vi "Noise Synthesis Test.vi"() -> ()   [LabVIEW 2015]
uses:
  Controls/Level XCtl/Level XCtl.xctl
  <vilib>/Analysis/5stat.llb/RMS (DBL).vi
  Top Level VIs/Stimulus-Set Level.vi
  Utility VIs/Math VIs/Linear to dB (scalar).vi
  Utility VIs/Math VIs/FFT x(t) to dB,Degrees (1D).vi
  <vilib>/Analysis/NI_AALPro.lvlib
panel:
  out "dB Vrms":dbl
  in  "Level":T2(xcontrol) caption="Level XCtl"
  in  "Slope Fmin (Hz)":dbl=500.0
  out "XY Graph":cluster{"Array":dbl[], "Array":dbl[]}(graph)
  out "Waveform Graph":dbl[](graph)
  out "error out":errorcluster
  in  "error in (no error)":errorcluster
  in  "Length (points)":i32=100000
  in  "Sampling rate (Hz)":dbl=50000.0
  in  "Max Frequency (Hz)":dbl=1000.0
  in  "Slope (dB/oct)":dbl=-3.0
  in  "Min Frequency (Hz)":dbl=100.0
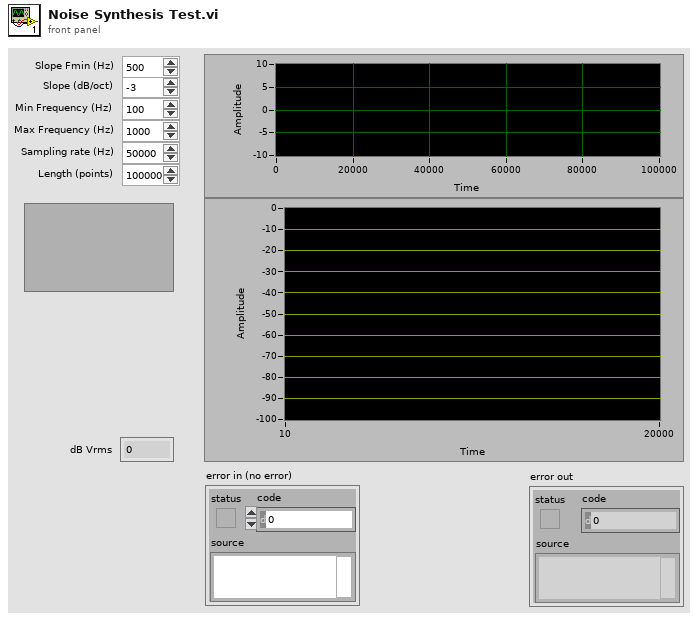
[diagram p1: front panel]
types:
  T1 = typedef "Level Units.ctl" = enum16{"dB atten", "dB SPL", "dB re 1 Vrms", "dB V/Hz½", "mW", "dB HL", "Volts", "dB mW"}
  T2 = cluster{"Level":dbl, "Units":T1, "Max":dbl, "Multiplier":dbl, "Cal File":path, "Cal":cluster{"Freq (Hz)":dbl[], "Mag (dB SPL)":dbl[], "Phase (deg)":dbl[]}}
  T3 = cluster{"Level":dbl, "Mode":T1, "Max":dbl, "Multiplier":dbl, "Cal File":path, "Cal":cluster{"Freq (Hz)":dbl[], "Mag (dB SPL)":dbl[], "Phase (deg)":dbl[]}}
  T4 = typedef "Level XCtl.xctl/Level Data.ctl" = cluster{"Level":dbl, "Units":T1, "Max":dbl, "Multiplier":dbl, "Cal File":path, "Cal":cluster{"Freq (Hz)":dbl[], "Mag (dB SPL)":dbl[], "Phase (deg)":dbl[]}}
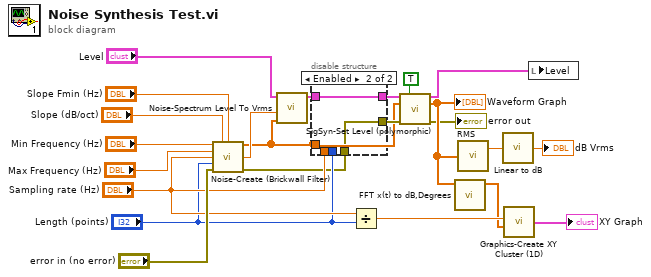
[diagram p0: block diagram]
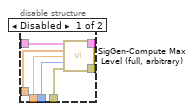
[diagram p2: hidden frame]
diagram:
  n1 = call "Noise-Create (Brickwall Filter).vi"("Min Frequency (Hz)"="Min Frequency (Hz)", "Slope (dB/oct)"="Slope (dB/oct)", "Slope Fmin (Hz)"="Slope Fmin (Hz)", "Max Frequency (Hz)"="Max Frequency (Hz)", "Sampling rate (Hz)"="Sampling rate (Hz)", "Length (points)"="Length (points)", "error in (no error)"="error in (no error)") -> ("Filtered Noise"=w2:dbl[], "dB Vrms of spectrum level = 0"=w14:dbl, "error out"=w4:errorcluster)  [unwired: 6 in]
  n2 = call "Noise-Spectrum Level To Vrms.vi"("Filtered Noise"=w2, "dB Vrms of spectrum level = 0"=w14, "Level In"="Level") -> ("Level Out"=w12:T3)  [unwired: 7 in, 1 out]
  n3 = disable-structure shown="Enabled" {
    disable-tunnel: w12 -> [w30 w32]
    disable-tunnel: [w29 w32] -> w11
    disable-tunnel: "Sampling rate (Hz)" -> [w28 _]
    disable-tunnel: "Length (points)" -> [w27 _]
    disable-tunnel: [w26 w31] -> w5
    disable-tunnel: w4 -> [w25 w31]
    disable-tunnel: w2 -> [w24 _]
    frame Disabled {
      n4 = call "SigGen-Compute Max Level (full, arbitrary).vi"("Level"=w30, "Y"=w24, "Sampling Rate (Hz)"=w28, "Npts"=w27, "error in (no error)"=w25) -> ("Level Out"=w29:T4, "error out"=w26:errorcluster)  [unwired: 8 in, 1 out]
    }
    frame Enabled {
    }
  }
  n5 = Divide(x="Sampling rate (Hz)", y="Length (points)") -> (x/y=w19:dbl)
  n6 = call-poly "SigSyn-Set Level (polymorphic).vi"("Level"=w11, "Apply multiplier? (F)"=TRUE, "Waveform in"=w2, "error in (no error)"=w5) -> ("Level out"=w1:T4, "Waveform out"=w8:dbl[], "error out"=→"error out":errorcluster)  [unwired: 7 in, 2 out]
  "Waveform Graph" <- w8
  n7 = call-poly "FFT x(t) to dB,Degrees.vi"("X"=w8) -> ("+Freq. Mag of FFT (dB rms)"=w18:dbl[])  [unwired: 8 in, 2 out]
  n8 = call-poly <vilib>:"RMS.vi"("X"=w8) -> ("rms value"=w7:dbl)  [unwired: 1 out]
  n9 = call-poly "Linear to dB.vi"("Linear"=w7) -> ("dB"=→"dB Vrms":dbl)
  n10 = call "Graphics-Create XY Cluster (1D).vi"("Array"=w18, "dx"=w19) -> ("XY cluster"=→"XY Graph":cluster{"Array":dbl[], "Array":dbl[]})  [unwired: 2 in]
  n11 = local write "Level"(w1) -> ()
